vi "qDCO.vi"(0 "System no.":i32=1 min=1 max=4 step=1, 2 "Axes to query":string[](array[string]), 3 "All axes?":bool, 4 "Axis identifier?":bool=TRUE, 5 "error in":errorcluster) -> (14 "Drift comp. mode?":bool[](array[boolean]), 19 "error out":errorcluster)   [LabVIEW 2026]
doc: "Returns drift compensation mode status of queried axes.\n\nE-516: If All axes = TRUE, then Axis identifier must be TRUE\n\nE-517, E-518: If All axes? = TRUE, then Axis identifier? can be FALSE\n\nE-816: All axes? = FALSE, only one axis per command allowed."
panel:
  # "Returns drift compensation mode status for queried axes."
  # "If all axes: use"
  # "Query"
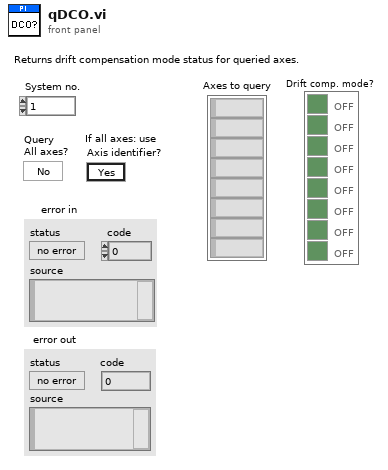
[diagram p1: front panel]
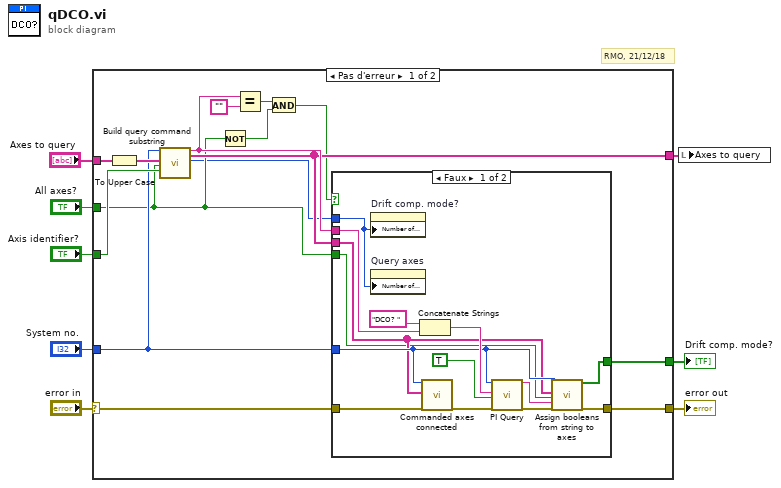
[diagram p0: block diagram]
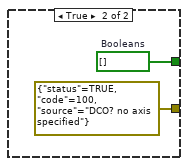
[diagram p2: hidden frame]
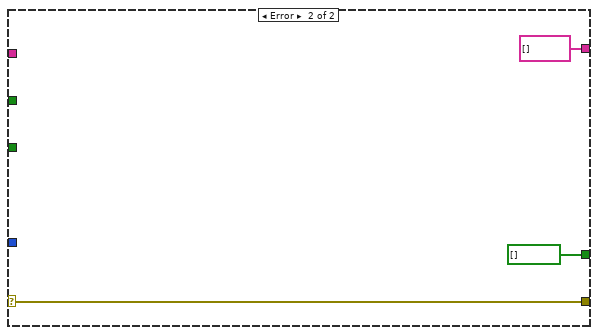
[diagram p3: hidden frame]
diagram:
  # "RMO, 21/12/18"
  n1 = case shown="Pas d'erreur" "error in" {
    selector: "error in" -> [w9 w40]
    tunnel: [w23 bool[] [] ("Booleans")] -> w8
    tunnel: "Axes to query" -> [w22 _]
    tunnel: [w11 w40] -> w6
    tunnel: "Axis identifier?" -> [w19 _]
    tunnel: "System no." -> [w17 _]
    tunnel: [w16 string[] [] ("Axes to query out")] -> w3
    tunnel: "All axes?" -> [w15 _]
    frame No Error {
      n2 = To Upper Case(1:w22) -> (0:w20:string[])
      n3 = call "Build query command substring.vi"("System no."=w17, "Axes to query in"=w20, "Query\nAll axes?"=w15, "For all axes: use\nAxis identifier?"=w19) -> ("Command substring"=w18:string, "Axes to query out"=w16:string[], "Number of rows"=w12:u32)  [unwired: 2 in, 11 out]
      n4 = Not(x=w15) -> (.not. x?=w13:bool)
      n5 = Equal?(x=w18, y="" ("x")) -> (x = y?=w14:bool)
      n6 = And(x=w14, y=w13) -> (x .and. y?=w10:bool)
      n7 = case shown="Faux" w10 {
        tunnel: [w34 w38] -> w23
        tunnel: w9 -> [w33 _]
        tunnel: w18 -> [w32 _]
        tunnel: w17 -> [w31 _]
        tunnel: w16 -> [w30 _]
        tunnel: w15 -> [w29 _]
        tunnel: w12 -> [w28 _]
        tunnel: [w26 errorcluster {"status"=TRUE, "code"=100, "source"="DCO? no axis specified"} ("error out")] -> w11
        frame False {
          n8 = property on="Drift comp. mode?" class="Tabl (strict)"("Number of Rows"=w28) -> ()  [unwired: 2 in, 2 out]
          n9 = property on="Query axes" class="Tabl (strict)"("Number of Rows"=w28) -> ()  [unwired: 2 in, 2 out]
          n10 = Concatenate Strings("DCO? ", w32) -> (w35:string)
          n11 = call "Commanded axes connected.vi"("System no."=w31, "Commanded axes"=w30, "error in"=w33) -> ("error out"=w27:errorcluster)  [unwired: 1 in, 15 out]
          n12 = call "PI Query.vi"("System no."=w31, "String to send"=w35, "Attach termination char.?"=TRUE ("Attach Linefeed?"), "error in"=w27) -> ("String read"=w24:string, "error out"=w25:errorcluster)  [unwired: 3 in, 11 out]
          n13 = call "Assign booleans from string to axes.vi"("System no."=w31, "Queried axes"=w30, "All axes queried?"=w29, "Input String"=w24, "error in"=w25) -> ("Booleans"=w34:bool[], "error out"=w26:errorcluster)  [unwired: 13 out]
        }
        frame True {
          w38 = bool[] []  # Booleans
        }
      }
    }
    frame Error {
    }
  }
  "error out" <- w6
  "Drift comp. mode?" <- w8
  n14 = local write "Axes to query"(w3) -> ()
